vi "simple_for_loop.vi"() -> ()   [LabVIEW 2021]
panel:
  out "x+y":i32[](array[numeric])
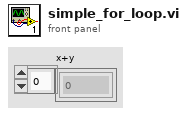
[diagram p1: front panel]
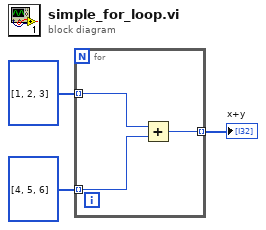
[diagram p0: block diagram]
diagram:
  n1 = for {
    tunnel: i32[] [1, 2, 3] -> [w6] mode=indexing
    tunnel: i32[] [4, 5, 6] -> [w5] mode=indexing
    tunnel: [w4] -> w1 mode=indexing
    n2 = Add(x=w6, y=w5) -> (x+y=w4:i32)
  }
  "x+y" <- w1
